vi "Decompress.vi"(9 "Block Data":string) -> (0 "Role Data":string)   [LabVIEW 2009, in "DSO1K.lvlib"]
doc: "The received data decompress image format"
uses:
  <instrlib>/DSO1K/DSO1K.lvlib
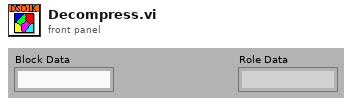
[diagram p1: front panel]
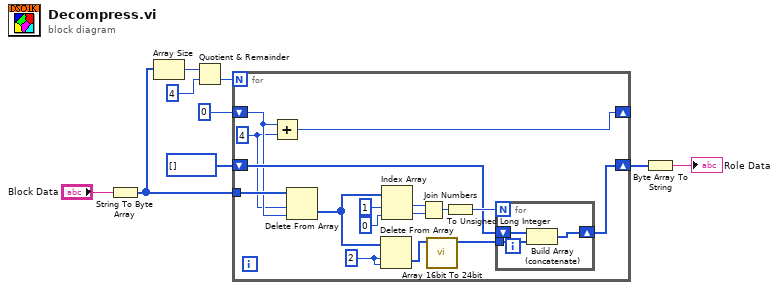
[diagram p0: block diagram]
diagram:
  n1 = String To Byte Array(string="Block Data") -> (unsigned byte array=w5:u8[])
  n2 = Array Size(array=w5) -> (size(s)=w9:i32)
  n3 = Quotient & Remainder(x=w9, y=4) -> (floor(x/y)=w8:i32)  [unwired: 1 out]
  n4 = for {
    N: w8 -> [_]
    shift-right: [w25] -> _
    shift-left: u32 0 -> [w11]
    tunnel: w5 -> [w15]
    shift-right: [w16] -> w3
    shift-left: u8[] [] -> [w17]
    w13 = 2 ("index")
    w10 = u32 4 ("y")
    n5 = Add(x=w11, y=w10) -> (x+y=w25:u32)
    n6 = Delete From Array(array=w15, length=w10, index=w11) -> (deleted portion=w14:u8[])  [unwired: 1 out]
    n7 = Delete From Array(array=w14, length=w13, index=w13) -> (deleted portion=w12:u8[])  [unwired: 1 out]
    n8 = Index Array(array=w14, index #1=1 ("index"), index #2=0 ("index")) -> (element #1=w20:u8, element #2=w21:u8)
    n9 = Join Numbers(hi=w20, lo=w21) -> ((hi.lo)=w24:u16)
    n10 = call <instrlib>:"Array 16bit To 24bit.vi"("Unsigned Byte Array"=w12) -> ("Appended Array"=w18:u8[])  [unwired: 10 in]
    n11 = To Unsigned Long Integer(number=w24) -> (unsigned 32bit integer=w19:u32)
    n12 = for {
      N: w19 -> [_]
      tunnel: w18 -> [w28]
      shift-right: [w26] -> w16
      shift-left: w17 -> [w27]
      n13 = Build Array (concatenate)(w27, w28) -> (w26:u8[])
    }
  }
  n14 = Byte Array To String(unsigned byte array=w3) -> (string=→"Role Data":string)
